vi "PrepareChannels.vi"() -> (0 "DO error out":errorcluster, 1 "DO task out":refnum<k21>, 2 "AO error out":errorcluster, 3 "AO task out":refnum<k21>, 5 "Waveform Graph":waveform(dbl)(graph))   [LabVIEW 2015]
uses:
  <vilib>/DAQmx/create/channels.llb/DAQmx Create Channel (AO-Voltage-Basic).vi
  <vilib>/DAQmx/configure/timing.llb/DAQmx Timing (Sample Clock).vi
  <vilib>/DAQmx/create/channels.llb/DAQmx Create Channel (DO-Digital Output).vi
panel:
  in  "DO Physical channels":tag="Dev1/port0/line0"
  in  "Sampling Rate (Hz)":dbl=100000.0
  in  "Amplitude (Volts)":dbl=1.0
  in  "Num Pulses":u32=1 min=1
  in  "Pulse Width (ms)":dbl=0.09
  in  "Pulse Type":enum16{"Monophasic", "Biphasic"}(ring)=enum."Biphasic"
  in  "AO Physical channels":tag="Dev1/ao0"
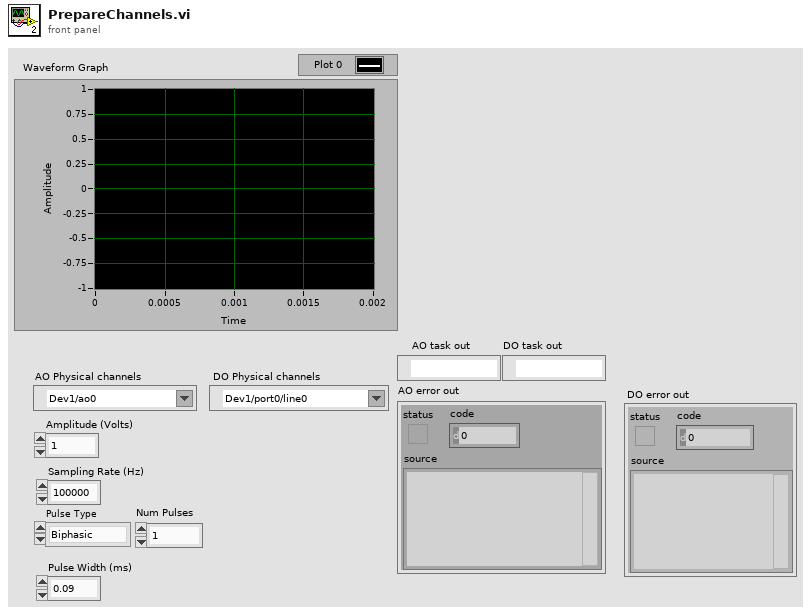
[diagram p1: front panel]
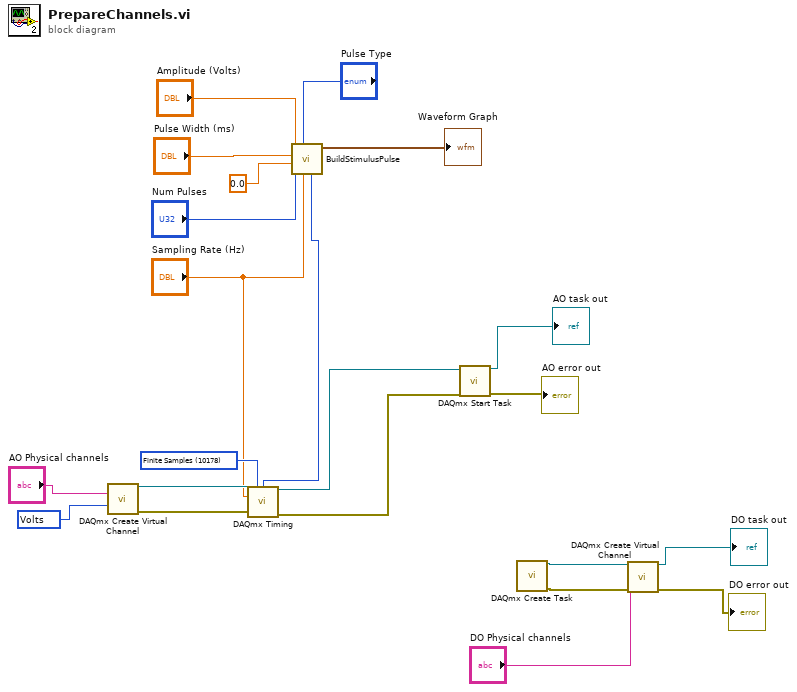
[diagram p0: block diagram]
diagram:
  w15 = 10178 items=["Finite Samples"=10178, "Continuous Samples"=10123, "Hardware Timed Single Point"=12522] ("sample mode")
  w22 = 10348 items=["Volts"=10348, "From Custom Scale"=10065] ("units")
  n1 = call-poly <vilib>:"DAQmx Create Virtual Channel.vi"("physical channels"="AO Physical channels", "units"=w22) -> ("task out"=w13:refnum<k21>, "error out"=w12:errorcluster)  [unwired: 12 in]
  n2 = call "BuildStimulusPulse.vi"("Sampling Rate (Hz)"="Sampling Rate (Hz)", "Pulse Type"="Pulse Type", "Num Pulses"="Num Pulses", "Inter-Pulse Interval (ms)"=0.0, "Pulse Width (ms)"="Pulse Width (ms)", "Amplitude (Volts)"="Amplitude (Volts)") -> ("Waveform Out"=→"Waveform Graph":waveform(dbl), "Final Array Size"=w14:i32)  [unwired: 3 in, 1 out]
  n3 = call-poly <vilib>:"DAQmx Timing.vi"("task/channels in"=w13, "sample mode"=w15, "samples per channel"=w14, "rate"="Sampling Rate (Hz)", "error in"=w12) -> ("task out"=w5:refnum<k21>, "error out"=w4:errorcluster)  [unwired: 9 in]
  n4 = call <vilib>:"DAQmx Start Task.vi"("task/channels in"=w5, "error in"=w4) -> ("task out"=→"AO task out":refnum<k21>, "error out"=→"AO error out":errorcluster)  [unwired: 12 in]
  n5 = call <vilib>:"DAQmx Create Task.vi"() -> ("task out"=w10:refnum<k21>, "error out"=w9:errorcluster)  [unwired: 14 in]
  n6 = call-poly <vilib>:"DAQmx Create Virtual Channel.vi"("task in"=w10, "lines"="DO Physical channels", "error in"=w9) -> ("task out"=→"DO task out":refnum<k21>, "error out"=→"DO error out":errorcluster)  [unwired: 11 in]
